vi "Server Handle Disconnect Message.vi"(8 "error in":errorcluster, 11 "state in":T1) -> (0 "error out":errorcluster, 3 "state out":T1)   [LabVIEW 2016, in "NI_CCC.lvlib"]
doc: "This VI deletes the groups created at the last configure. This prevents memory leakage of old group data in the CVT group memory."
uses:
  NI_CCC.lvlib
  Server State.ctl
  <vilib>/NI/Current Value Table/FGVs/Group Memory.vi
  <vilib>/NI/Current Value Table/Current Value Table.lvlib
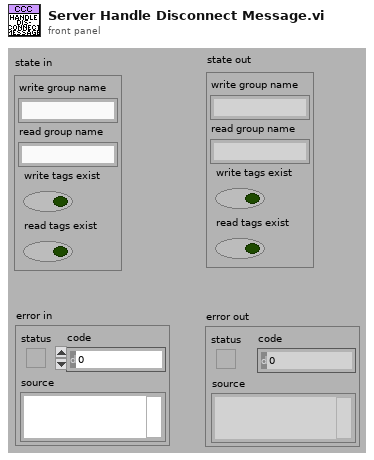
[diagram p1: front panel]
types:
  T1 = typedef "NI_CCC.lvlib/Server State.ctl" = cluster{"write group name":string, "read group name":string, "write tags exist":bool, "read tags exist":bool}
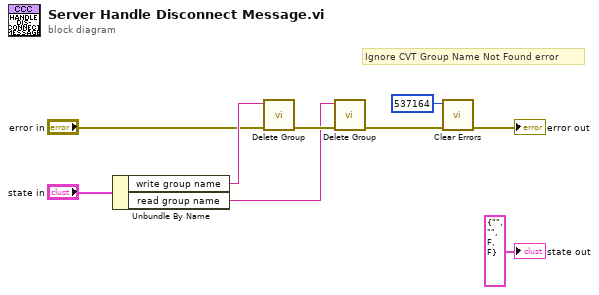
[diagram p0: block diagram]
diagram:
  # "Ignore CVT Group Name Not Found error"
  n1 = Unbundle By Name("state in") -> ("write group name"=w7:string, "read group name"=w5:string)
  n2 = call <vilib>:"Delete Group.vi"("error in (no error)"="error in", "Group"=w7) -> ("error out"=w6:errorcluster)  [unwired: 9 in]
  n3 = call <vilib>:"Delete Group.vi"("error in (no error)"=w6, "Group"=w5) -> ("error out"=w2:errorcluster)  [unwired: 9 in]
  n4 = call <vilib>:"Clear Errors.vi"("error in (no error)"=w2, "specific error code to clear (0: all)"=537164) -> ("error out"=→"error out":errorcluster)  [unwired: 4 in, 1 out]
  "state out" <- T1 {"write group name"="", "read group name"="", "write tags exist"=FALSE, "read tags exist"=FALSE} ("state out")
